vi "oprea edited code.vi"   [LabVIEW 2018]
types:
  T1 = typedef "IMAQ Image.ctl" = refnum<image>
  T2 = cluster{"Corners":cluster{"X":sgl, "Y":sgl}[], "Orientation (degrees)":dbl, "Width":dbl, "Height":dbl, "Score":dbl}[]
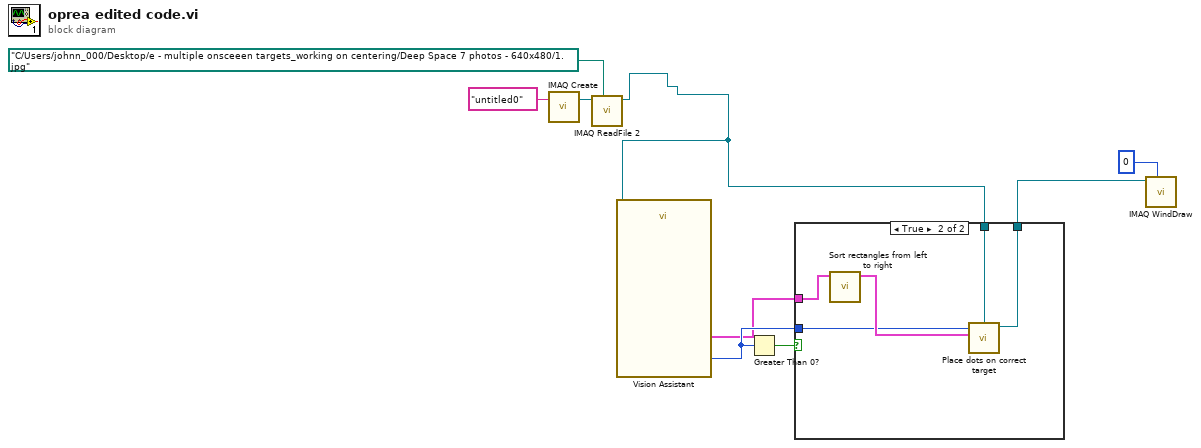
[diagram p0: block diagram]
diagram:
  n1 = call "IMAQ Create"("Image Name"="untitled0") -> ("New Image"=w7:T1)  [unwired: 4 in, 1 out]
  n2 = call "IMAQ ReadFile 2"("File Path"=path "C:/Users/johnn_000/Desktop/e - multiple onsceeen targets_working on centering/Deep Space 7 photos - 640x480/1.jpg", "Image"=w7) -> ("Image Out"=w1:T1)  [unwired: 5 in, 4 out]
  n3 = call "Vision Assistant"("Image In"=w1) -> ("Number of Matches (Shape Detection 1)"=w8:i32, "Rectangles Calibrated (Shape Detection 1)"=w4:T2)  [unwired: 23 in, 2 out]
  n4 = Greater Than 0?(x=w8) -> (x > 0?=w9:bool)
  n5 = case shown="True" w9 {
    tunnel: [w10 w15] -> w2
    tunnel: w4 -> [_ w13]
    tunnel: w8 -> [_ w12]
    tunnel: w1 -> [w10 w11]
    frame False {
    }
    frame True {
      n6 = call "Sort rectangles from left to right.vi"("Rectangles (Calibrated) IN"=w13) -> ("Rectangles (Calibrated) OUT"=w14:T2)  [unwired: 10 in]
      n7 = call "Place dots on correct target.vi"("# rectangles"=w12, "Rectangles (Calibrated)"=w14, "Image"=w11) -> ("Image Out"=w15:T1)  [unwired: 8 in]
    }
  }
  n8 = call "IMAQ WindDraw"("Window Number (0...15)"=0, "Image"=w2) -> ()  [unwired: 8 in, 2 out]
